vi "Keyence.Global.vi"() -> ()   [LabVIEW 2016]
uses:
  Keyence.CodeDetails.ctl
  Keyence.Data.Status.ctl
  Keyence.Data.Status.State.ctl
  Keyence.Data.Sets.ctl
panel:
  out "OrderScanner.Code":T1
  out "OrderScanner.Status":T2={"State"=enum."Init", "Ref"=refnum, "Bank"=0, "Version"="", "Model"="", "EndTS"=timestamp(0 s since 1904-01-01), "ImgPath"=path "", "Tuned"=FALSE}
  in  "OrderScanner.Sets":T4
  out "Keyence.Abort":bool
  out "Keyence.Stop":bool
  in  "ProdScanner.Sets":T4
  out "ProdScanner.Status":T2={"State"=enum."Init", "Ref"=refnum, "Bank"=0, "Version"="", "Model"="", "EndTS"=timestamp(0 s since 1904-01-01), "ImgPath"=path "", "Tuned"=FALSE}
  out "ProdScanner.Code":T1
  out "LogPath":path=path "C:/SOFTWARE/logs/scanner"
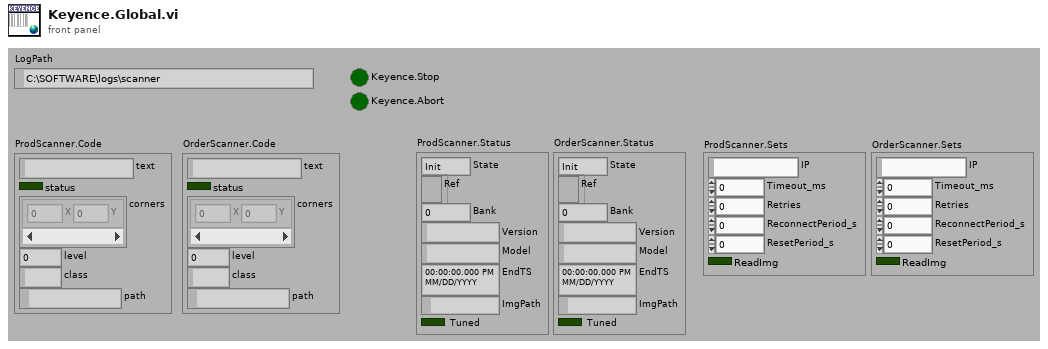
[diagram p1: front panel]
types:
  T1 = typedef "Keyence.CodeDetails.ctl" = cluster{"text":string, "status":bool, "corners":cluster{"X":i32, "Y":i32}[], "level":u8, "class":string, "path":path}
  T2 = typedef "Keyence.Data.Status.ctl" = cluster{"State":T3, "Ref":refnum<k5>, "Bank":u8, "Version":string, "Model":string, "EndTS":timestamp, "ImgPath":path, "Tuned":bool}
  T3 = typedef "Keyence.Data.Status.State.ctl" = enum16{"First", "Init", "Reset", "Idle", "Scan", "Tune"}
  T4 = typedef "Keyence.Data.Sets.ctl" = cluster{"IP":string, "Timeout_ms":i32, "Retries":i32, "ReconnectPeriod_s":i32, "ResetPeriod_s":i32, "ReadImg":bool}
diagram:
